vi "DeepU Front Panel.vi"() -> ()   [LabVIEW 2019, in "Results.lvlib" / "DeepU Results.lvclass"]
uses:
  DeepU Results.lvclass
  DeepU Results.lvclass/DeepU Results.ctl
  Test Stands/DeepU/DeepU Test Stand.lvclass
panel:
  out "TC Unit 2":string
  in  "Std Dev":bool
  out "Numeric":dbl=1.0
  in  "x std_dev":dbl=3.0 min=2.0 max=3.0 step=1.0 format="%#.0f"
  out "dp PD-23X 4 std":dbl caption="PDX 4 std" format="%#10.0f"
  out "dp PD-23X 3 std":dbl caption="PDX 3 std" format="%#10.0f"
  out "dp PD-23X 2 std":dbl caption="PDX 2 std" format="%#10.0f"
  out "dp PD-23X 1 std":dbl caption="PDX 1 std" format="%#10.0f"
  out "dp PD-23 5 std":dbl caption="PD 5 std" format="%10.0f"
  out "dp PD-23 2 std":dbl caption="PD 2 std" format="%10.0f"
  out "dp PD-23 3 std":dbl caption="PD 3 std" format="%10.0f"
  out "dp PD-23 4 std":dbl caption="PD 4 std" format="%10.0f"
  out "dp PD-23 1 std":dbl caption="PD 1 std" format="%10.0f"
  out "J 3 std":dbl format="%10.0f"
  out "J 1 std":dbl format="%10.0f"
  out "J 2 std":dbl format="%10.0f"
  out "Fan Temp":dbl format="%#.1f"
  out "Fan Temperature":dbl(slide) scale=0.0..200.0
  out "Inv Temp":u16 caption="Inv Temp, C"
  out "Fan rpm":u16
  out "Fan I":dbl caption="Fan I, A" format="%.1f"
  out "Fan Const":bool=TRUE
  out "In range?":bool
  out "Inlet Pressure":dbl(knob) caption="Bed Pressure, kPa (g)" scale=0.0..20.0
  out "TC Unit":string
  out "pa 2":dbl caption="p bed" format="%10.0f"
  out "pa 1":dbl caption="pb" format="%10.0f"
  out "dp J 3":dbl format="%10.0f"
  out "dp J 1":dbl format="%10.0f"
  out "dp J 2":dbl format="%10.0f"
  out "dp PD-23X 3":dbl caption="PDX 3" format="%#10.0f"
  out "dp PD-23X 1":dbl caption="PDX 1" format="%#10.0f"
  out "dp PD-23X 2":dbl caption="PDX 2" format="%#10.0f"
  out "dp PD-23X 4":dbl caption="PDX 4" format="%#10.0f"
  out "Gas Humidity":dbl caption="%RH" format="%#.1f"
  out "T2":dbl format="%#5.1f"
  out "T1":dbl format="%#5.1f"
  out "Adjusted":bool
  in  "Gas Flow SP":sgl caption="Gas Flow" min=0 max=372 step=1
  in  "auto Flow":bool
  in  "Fan Out Ctrl":dbl caption="Fan Output (2 - 200 Hz)" min=0.0 max=200.0 step=1.0 format="%6.2f"
  in  "Gas Speed SP":sgl caption="Gas Speed" min=0 max=300 step=1
  out "Fan Output":dbl(slide) scale=0.0..100.0
  in  "auto":bool
  out "Gas Flow":sgl caption="Gas Flow, l/s" format="%.1f"
  out "Gas Speed":sgl caption="Gas speed" format="%10.2f"
  out "dp PD-23 4":dbl caption="PD 4" format="%10.0f"
  out "dp PD-23 2":dbl caption="PD 2" format="%10.0f"
  out "dp PD-23 1":dbl caption="PD 1" format="%10.0f"
  out "dp PD-23 3":dbl caption="PD 3" format="%10.0f"
  out "dp PD-23 5":dbl caption="PD 5" format="%10.0f"
  # "Pressure in Pa"
  # "mean"
  # "Automatic"
  # "mean"
  # "Manual"
  # "std_dev"
  # "%"
  # "C"
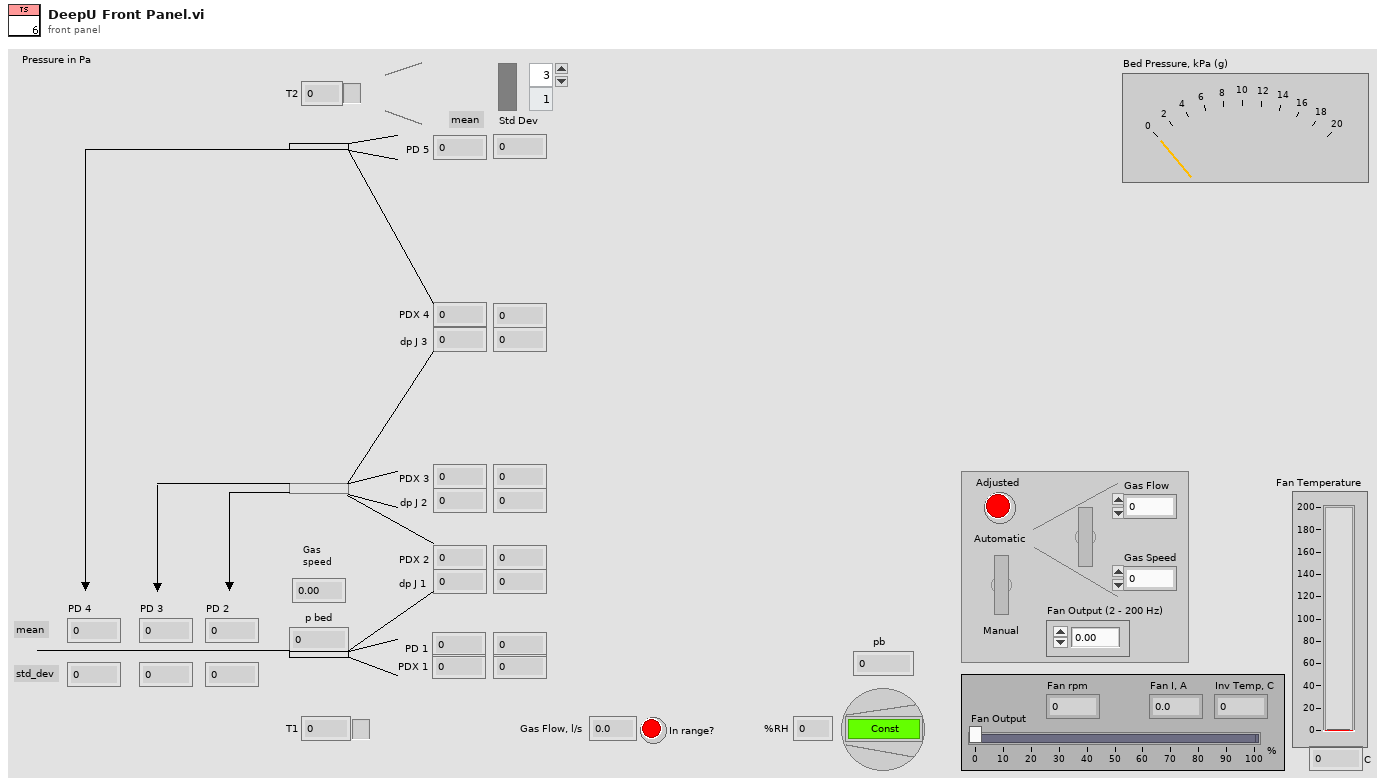
[diagram p1: front panel]
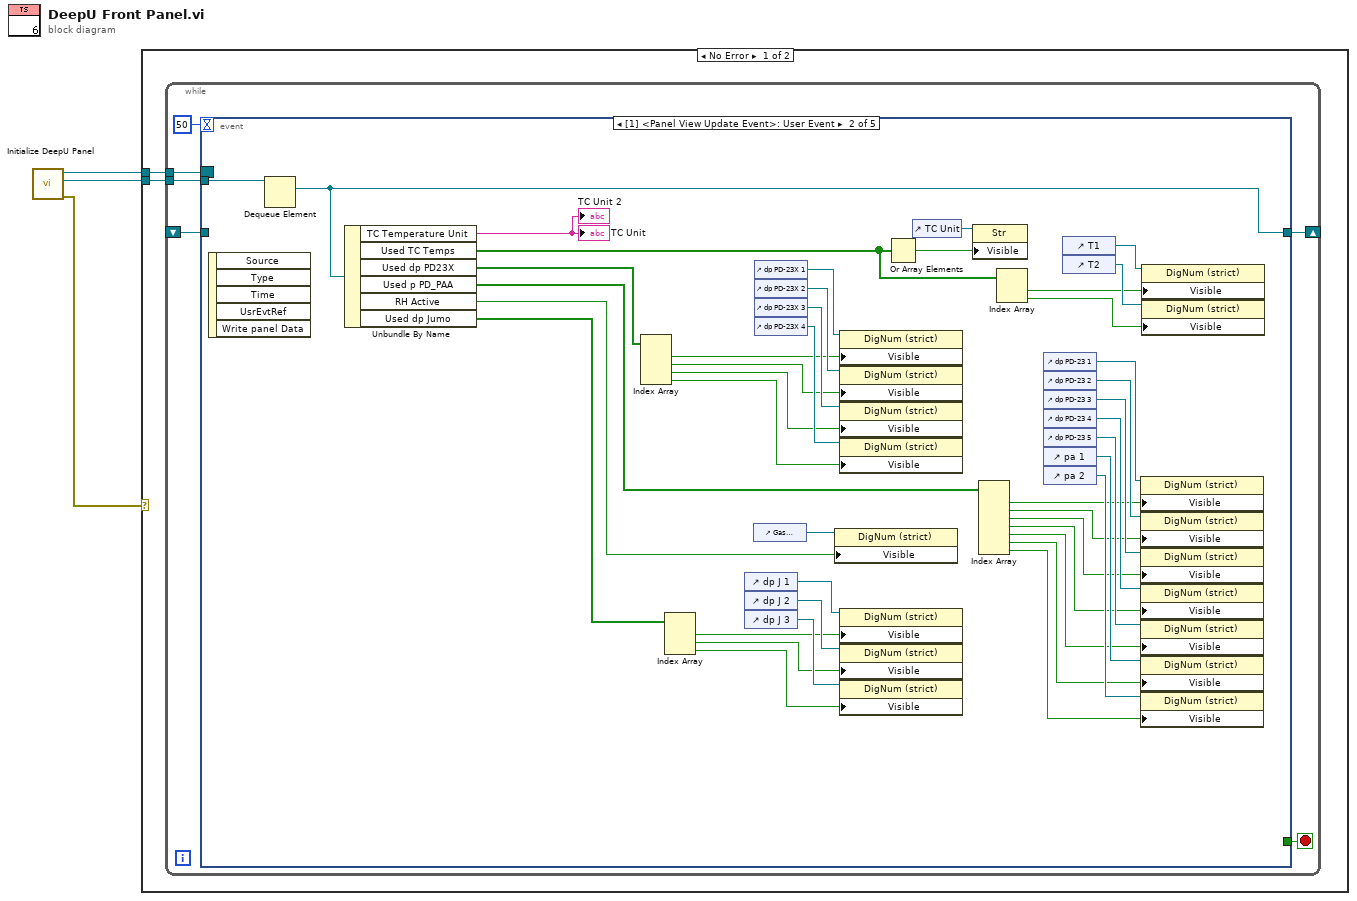
[diagram p0: block diagram]
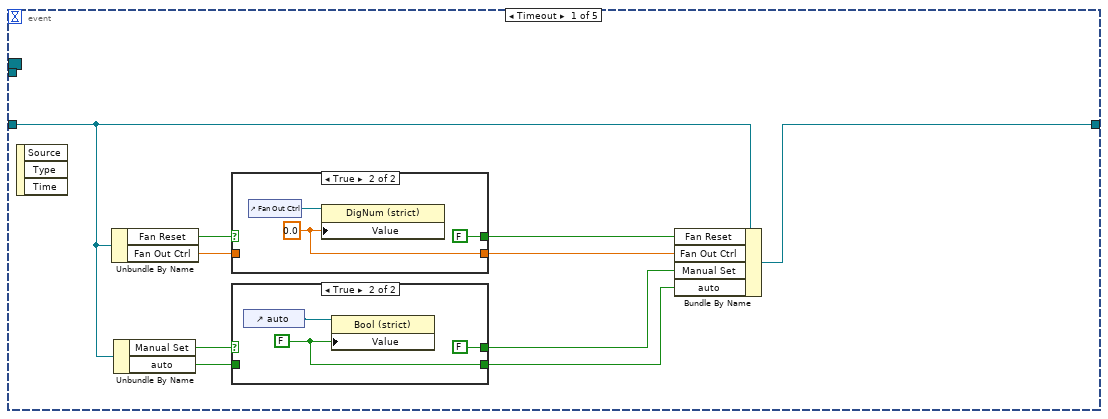
[diagram p2: hidden frame]
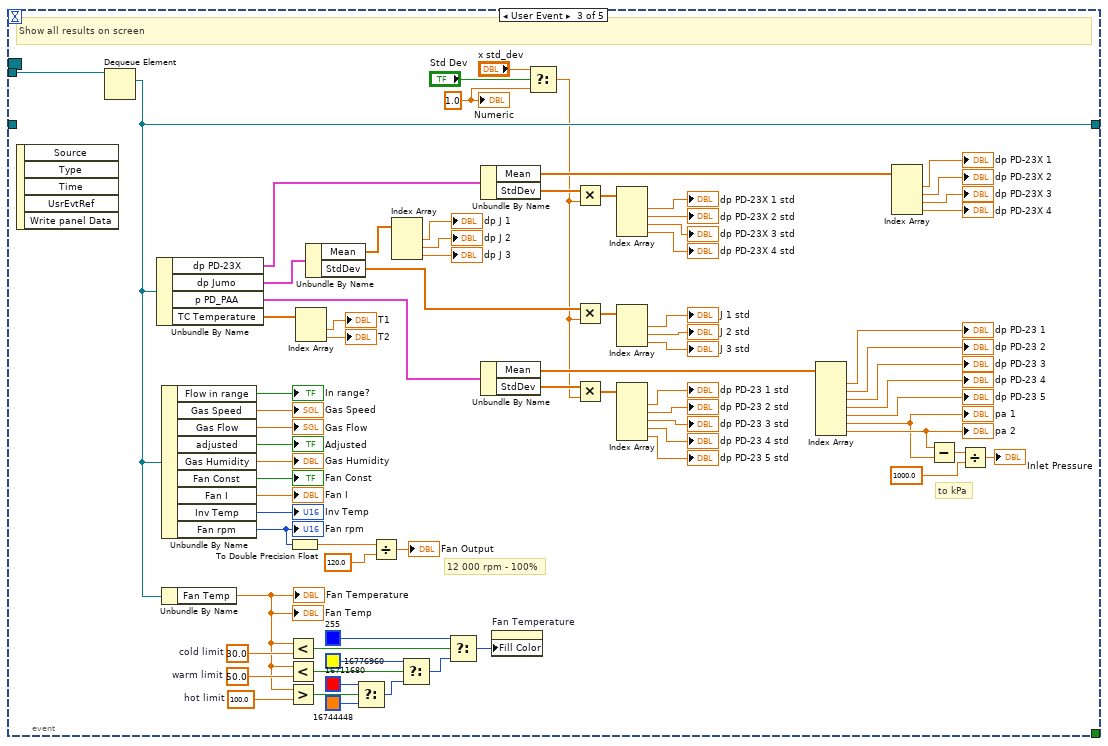
[diagram p5: hidden frame]
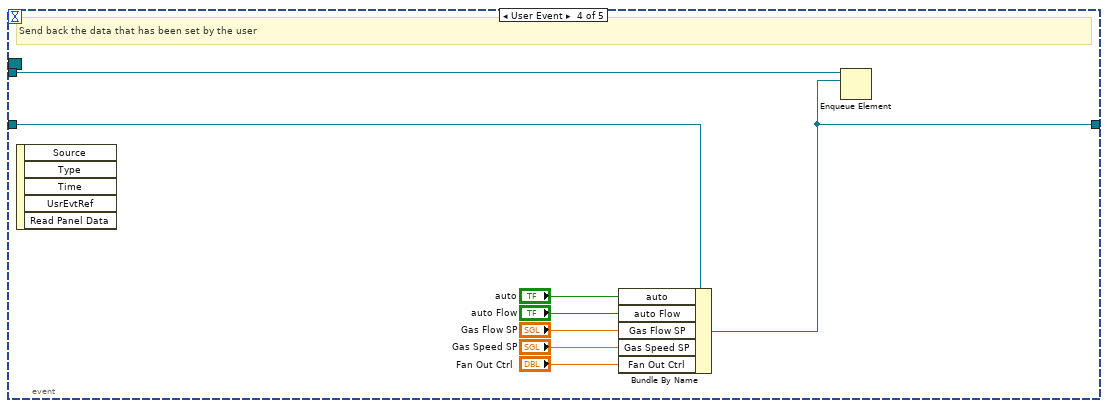
[diagram p6: hidden frame]
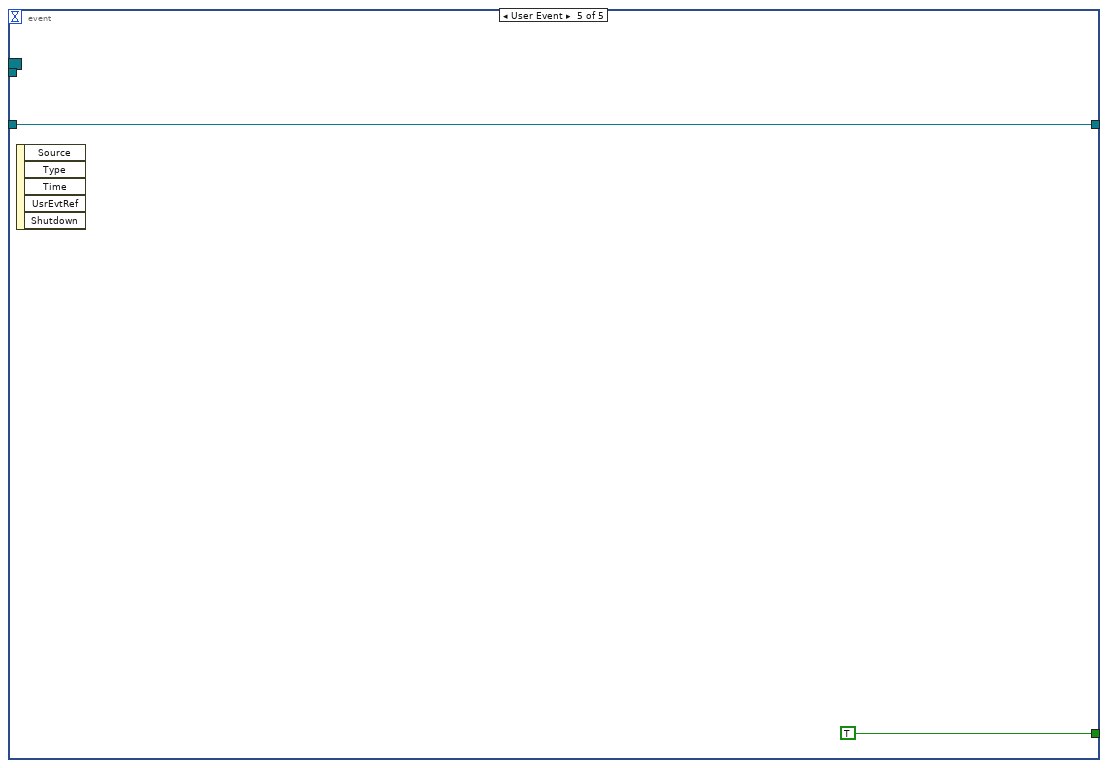
[diagram p7: hidden frame]
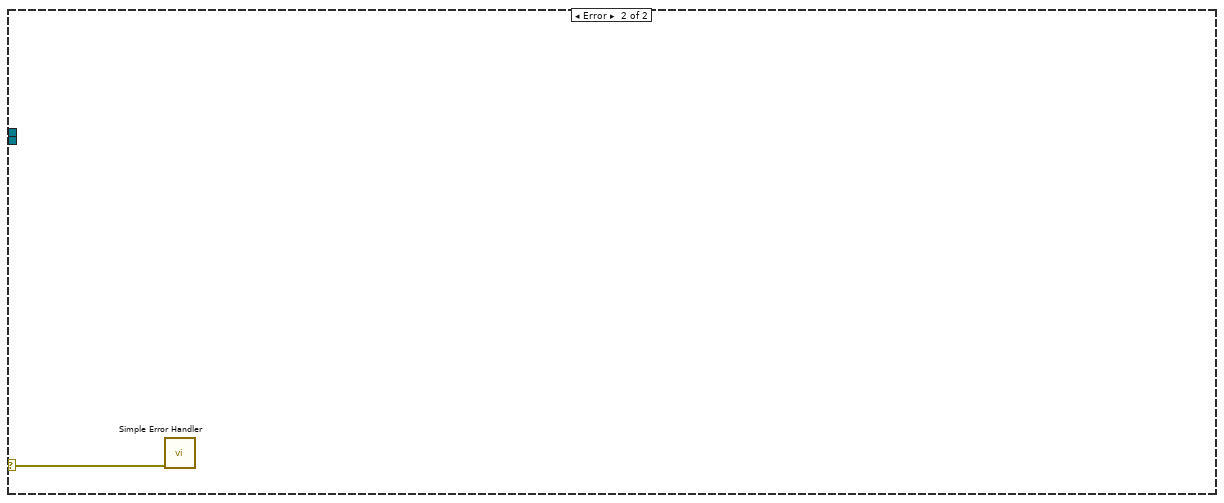
[diagram p8: hidden frame]
diagram:
  n1 = call "Initialize DeepU Panel.vi"() -> ("error out"=w3:errorcluster, "DeepU Results queue out"=w1:refnum<queue>, "Event Registration Refnum"=w2:refnum<event-registration>)  [unwired: 9 in]
  n2 = case shown="No Error" w3 {
    selector: w3 -> [_ w161]
    tunnel: w2 -> [w5 _]
    tunnel: w1 -> [w4 _]
    frame No Error {
      n3 = while {
        tunnel: w5 -> [w10]
        tunnel: w4 -> [w9]
        shift-right: [w7] -> _
        shift-left: _ -> [w6]
        stop <- w11 stop-if-true
        n4 = event shown="[1] <Panel View Update Event>: User Event" {
          selector: w10 -> [_ _ _ _ _]
          dyn-events: _ -> [_ _ _ _ _]
          timeout: 50 -> [_ _ _ _ _]
          tunnel: [_ _ _ _ TRUE] -> w11
          tunnel: w9 -> [_ w74 w150 w158 _]
          tunnel: [w21 w73 w132 w156 w159] -> w7
          tunnel: w6 -> [w16 _ _ w157 w159]
          event Timeout {
            n5 = event-data() -> ()  [unwired: 1 in, 3 out]
            n6 = Unbundle By Name(w16) -> ("Fan Reset"=w20:bool, "Fan Out Ctrl"=w19:dbl)
            n7 = Unbundle By Name(w16) -> ("Manual Set"=w15:bool, "auto"=w14:bool)
            n8 = case shown="True" w20 {
              selector: w20 -> [w27 _]
              tunnel: w19 -> [w28 _]
              tunnel: [w28 w29] -> w17
              tunnel: [w27 FALSE] -> w18
              frame False {
              }
              frame True {
                w29 = 0.0 ("t")
                n9 = control-ref of="Fan Out Ctrl"() -> (w31:refnum<vi>)
                n10 = property class="DigNum (strict)"(reference=w31, "Value"=w29) -> ()  [unwired: 1 in, 2 out]
              }
            }
            n11 = case shown="True" w15 {
              selector: w15 -> [w22 _]
              tunnel: w14 -> [w23 _]
              tunnel: [w23 w24] -> w12
              tunnel: [w22 FALSE] -> w13
              frame False {
              }
              frame True {
                w24 = FALSE
                n12 = control-ref of="auto"() -> (w25:refnum<vi>)
                n13 = property class="Bool (strict)"(reference=w25, "Value"=w24) -> ()  [unwired: 1 in, 2 out]
              }
            }
            n14 = Bundle By Name(cluster=w16, "Fan Reset"=w18, "Fan Out Ctrl"=w17, "Manual Set"=w13, "auto"=w12) -> (w21:refnum<class "DeepU Results.lvclass">)
          }
          event User Event {
            n15 = event-data() -> ()  [unwired: 1 in, 5 out]
            n16 = Dequeue Element(queue=w74) -> (element=w73:refnum<class "DeepU Results.lvclass">)  [unwired: 2 in, 3 out]
            n17 = Unbundle By Name(w73) -> ("TC Temperature Unit"=→"TC Unit" →"TC Unit 2":string, "Used TC Temps"=w69:bool[], "Used dp PD23X"=w64:bool[], "Used p PD_PAA"=w52:bool[], "RH Active"=w41:bool, "Used dp Jumo"=w37:bool[])
            n18 = Index Array(array=w64) -> (element #1=w63:bool, element #2=w62:bool, element #3=w61:bool, element #4=w60:bool)  [unwired: 4 in]
            n19 = Index Array(array=w37) -> (element #1=w36:bool, element #2=w35:bool, element #3=w34:bool)  [unwired: 3 in]
            n20 = control-ref of="dp J 1"() -> (w40:refnum<vi>)
            n21 = control-ref of="dp J 2"() -> (w39:refnum<vi>)
            n22 = control-ref of="dp J 3"() -> (w38:refnum<vi>)
            n23 = control-ref of="Gas Humidity"() -> (w44:refnum<vi>)
            n24 = control-ref of="dp PD-23X 1"() -> (w68:refnum<vi>)
            n25 = control-ref of="dp PD-23X 2"() -> (w67:refnum<vi>)
            n26 = control-ref of="dp PD-23X 3"() -> (w66:refnum<vi>)
            n27 = control-ref of="dp PD-23X 4"() -> (w65:refnum<vi>)
            n28 = property class="DigNum (strict)"(reference=w44, "Visible"=w41) -> ()  [unwired: 1 in, 2 out]
            n29 = property class="DigNum (strict)"(reference=w68, "Visible"=w63) -> ()  [unwired: 1 in, 2 out]
            n30 = property class="DigNum (strict)"(reference=w67, "Visible"=w62) -> ()  [unwired: 1 in, 2 out]
            n31 = property class="DigNum (strict)"(reference=w66, "Visible"=w61) -> ()  [unwired: 1 in, 2 out]
            n32 = property class="DigNum (strict)"(reference=w65, "Visible"=w60) -> ()  [unwired: 1 in, 2 out]
            n33 = property class="DigNum (strict)"(reference=w40, "Visible"=w36) -> ()  [unwired: 1 in, 2 out]
            n34 = property class="DigNum (strict)"(reference=w39, "Visible"=w35) -> ()  [unwired: 1 in, 2 out]
            n35 = property class="DigNum (strict)"(reference=w38, "Visible"=w34) -> ()  [unwired: 1 in, 2 out]
            n36 = Or Array Elements(Boolean array=w69) -> (logical OR=w43:bool)
            n37 = control-ref of="TC Unit"() -> (w72:refnum<vi>)
            n38 = property class="Str"(reference=w72, "Visible"=w43) -> ()  [unwired: 1 in, 2 out]
            n39 = Index Array(array=w52) -> (element #1=w51:bool, element #2=w45:bool, element #3=w46:bool, element #4=w47:bool, element #5=w48:bool, element #6=w49:bool, element #7=w50:bool)  [unwired: 7 in]
            n40 = Index Array(array=w69) -> (element #1=w42:bool, element #2=w33:bool)  [unwired: 2 in]
            n41 = control-ref of="dp PD-23 1"() -> (w59:refnum<vi>)
            n42 = control-ref of="dp PD-23 2"() -> (w58:refnum<vi>)
            n43 = control-ref of="dp PD-23 3"() -> (w57:refnum<vi>)
            n44 = control-ref of="dp PD-23 4"() -> (w56:refnum<vi>)
            n45 = control-ref of="dp PD-23 5"() -> (w55:refnum<vi>)
            n46 = control-ref of="pa 1"() -> (w54:refnum<vi>)
            n47 = control-ref of="pa 2"() -> (w53:refnum<vi>)
            n48 = control-ref of="T1"() -> (w70:refnum<vi>)
            n49 = control-ref of="T2"() -> (w71:refnum<vi>)
            n50 = property class="DigNum (strict)"(reference=w59, "Visible"=w51) -> ()  [unwired: 1 in, 2 out]
            n51 = property class="DigNum (strict)"(reference=w58, "Visible"=w45) -> ()  [unwired: 1 in, 2 out]
            n52 = property class="DigNum (strict)"(reference=w57, "Visible"=w46) -> ()  [unwired: 1 in, 2 out]
            n53 = property class="DigNum (strict)"(reference=w56, "Visible"=w47) -> ()  [unwired: 1 in, 2 out]
            n54 = property class="DigNum (strict)"(reference=w55, "Visible"=w48) -> ()  [unwired: 1 in, 2 out]
            n55 = property class="DigNum (strict)"(reference=w54, "Visible"=w49) -> ()  [unwired: 1 in, 2 out]
            n56 = property class="DigNum (strict)"(reference=w53, "Visible"=w50) -> ()  [unwired: 1 in, 2 out]
            n57 = property class="DigNum (strict)"(reference=w70, "Visible"=w42) -> ()  [unwired: 1 in, 2 out]
            n58 = property class="DigNum (strict)"(reference=w71, "Visible"=w33) -> ()  [unwired: 1 in, 2 out]
          }
          event User Event {
            w77 = 1.0 ("Numeric")
            w130 = 100.0  # hot limit
            w134 = 50.0  # warm limit
            w136 = 30.0  # cold limit
            # "to kPa"
            # "12 000 rpm - 100%"
            # "Show all results on screen"
            n59 = event-data() -> ()  [unwired: 1 in, 5 out]
            n60 = Dequeue Element(queue=w150) -> (element=w132:refnum<class "DeepU Results.lvclass">)  [unwired: 2 in, 3 out]
            n61 = Unbundle By Name(w132) -> ("dp PD-23X"=w146:cluster{"Mean":dbl[], "StdDev":dbl[]}, "dp Jumo"=w118:cluster{"Mean":dbl[], "StdDev":dbl[]}, "p PD_PAA"=w86:cluster{"Mean":dbl[], "StdDev":dbl[]}, "TC Temperature"=w85:dbl[])
            n62 = Unbundle By Name(w132) -> ("Flow in range"=→"In range?":bool, "Gas Speed"=→"Gas Speed":sgl, "Gas Flow"=→"Gas Flow":sgl, "adjusted"=→"Adjusted":bool, "Gas Humidity"=→"Gas Humidity":dbl, "Fan Const"=→"Fan Const":bool, "Fan I"=→"Fan I":dbl, "Inv Temp"=→"Inv Temp":u16, "Fan rpm"=w138:u16)
            "Fan rpm" <- w138
            n63 = Unbundle By Name(w132) -> ("Fan Temp"=w122:dbl)
            "Fan Temperature" <- w122
            "Fan Temp" <- w122
            n64 = Less?(x=w122, y=w136) -> (x < y?=w135:bool)
            n65 = Less?(x=w122, y=w134) -> (x < y?=w133:bool)
            n66 = Greater?(x=w122, y=w130) -> (0:w131:bool)
            n67 = To Double Precision Float(number=w138) -> (double precision float=w137:dbl)
            n68 = Index Array(array=w85) -> (element #1=→"T1":dbl, element #2=→"T2":dbl)  [unwired: 2 in]
            n69 = Unbundle By Name(w118) -> ("Mean"=w117:dbl[], "StdDev"=w82:dbl[])
            n70 = Select(t=u32 16711680 ("Fill Color"), s=w131, f=u32 16744448 ("Fill Color")) -> (s? t:f=w124:u32)
            n71 = Divide(x=w137, y=120.0) -> (x/y=→"Fan Output":dbl)
            n72 = Index Array(array=w117) -> (element #1=→"dp J 1":dbl, element #2=→"dp J 2":dbl, element #3=→"dp J 3":dbl)  [unwired: 3 in]
            n73 = Select(t=u32 16776960 ("Fill Color"), s=w133, f=w124) -> (s? t:f=w129:u32)
            n74 = Select(t=u32 255 ("Fill Color"), s=w135, f=w129) -> (s? t:f=w123:u32)
            n75 = Unbundle By Name(w146) -> ("Mean"=w102:dbl[], "StdDev"=w80:dbl[])
            n76 = Unbundle By Name(w86) -> ("Mean"=w101:dbl[], "StdDev"=w84:dbl[])
            n77 = property on="Fan Temperature" class="Slide (strict)"("Fill Color"=w123) -> ()  [unwired: 2 in, 2 out]
            n78 = Select(t="x std_dev", s="Std Dev", f=w77) -> (s? t:f=w75:dbl)
            n79 = Multiply(x=w80, y=w75) -> (x*y=w79:dbl[])
            n80 = Multiply(x=w82, y=w75) -> (x*y=w81:dbl[])
            n81 = Multiply(x=w84, y=w75) -> (x*y=w83:dbl[])
            n82 = Index Array(array=w79) -> (element #1=→"dp PD-23X 1 std":dbl, element #2=→"dp PD-23X 2 std":dbl, element #3=→"dp PD-23X 3 std":dbl, element #4=→"dp PD-23X 4 std":dbl)  [unwired: 4 in]
            n83 = Index Array(array=w81) -> (element #1=→"J 1 std":dbl, element #2=→"J 2 std":dbl, element #3=→"J 3 std":dbl)  [unwired: 3 in]
            n84 = Index Array(array=w83) -> (element #1=→"dp PD-23 1 std":dbl, element #2=→"dp PD-23 2 std":dbl, element #3=→"dp PD-23 3 std":dbl, element #4=→"dp PD-23 4 std":dbl, element #5=→"dp PD-23 5 std":dbl)  [unwired: 5 in]
            n85 = Index Array(array=w101) -> (element #1=→"dp PD-23 1":dbl, element #2=→"dp PD-23 2":dbl, element #3=→"dp PD-23 3":dbl, element #4=→"dp PD-23 4":dbl, element #5=→"dp PD-23 5":dbl, element #6=w99:dbl, element #7=w100:dbl)  [unwired: 7 in]
            "pa 1" <- w99
            "pa 2" <- w100
            n86 = Index Array(array=w102) -> (element #1=→"dp PD-23X 1":dbl, element #2=→"dp PD-23X 2":dbl, element #3=→"dp PD-23X 3":dbl, element #4=→"dp PD-23X 4":dbl)  [unwired: 4 in]
            n87 = Subtract(x=w100, y=w99) -> (x-y=w121:dbl)
            n88 = Divide(x=w121, y=1000.0) -> (x/y=→"Inlet Pressure":dbl)
            "Numeric" <- w77
          }
          event User Event {
            # "Send back the data that has been set by the user"
            n89 = event-data() -> ()  [unwired: 1 in, 5 out]
            n90 = Bundle By Name(cluster=w157, "auto"="auto", "auto Flow"="auto Flow", "Gas Flow SP"="Gas Flow SP", "Gas Speed SP"="Gas Speed SP", "Fan Out Ctrl"="Fan Out Ctrl") -> (w156:refnum<class "DeepU Results.lvclass">)
            n91 = Enqueue Element(queue=w158, element=w156) -> ()  [unwired: 2 in, 3 out]
          }
          event User Event {
            n92 = event-data() -> ()  [unwired: 1 in, 5 out]
          }
        }
      }
    }
    frame Error {
      n93 = call <vilib>:"Simple Error Handler.vi"("error in (no error)"=w161) -> ()  [unwired: 4 in, 5 out]
    }
  }
